vi "Save_file_txt_fifo.vi"(10 "传递队列":refnum<queue>, 11 "notifier":refnum<notifier>) -> ()   [LabVIEW 2012]
uses:
  <vilib>/GPower/VIRegister/Library/SubVIs/FindRegisterData.vi
  <vilib>/GPower/VIRegister/Library/SubVIs/WriteSub.vi
  <vilib>/GPower/Error/Library/FilterCodes.vi
  <vilib>/GPower/Error/Library/Filter/FilterMulti.vi
  <vilib>/GPower/VIRegister/Library/QManager/GetRegisterData.vi
  <vilib>/GPower/Error/Library/SetError.vi
  <vilib>/GPower/Error/Library/SplitAppended.vi
  <vilib>/GPower/VIRegister/Library/QManager/QManagerAction.vi
  <vilib>/GPower/Error/Library/ErrorType.vi
  <vilib>/GPower/Error/Library/SubVIs/ExplanationToError.vi
  <vilib>/GPower/VIRegister/Library/QManager/GetQName.vi
  <vilib>/GPower/VIRegister/Library/QManager/StartQManager.vi
  <vilib>/Utility/error.llb/Trim Whitespace.vi
  <vilib>/dlg_ctls.llb/Space Constant.vi
  <vilib>/Utility/error.llb/Error Code Database.vi
  <vilib>/GPower/Error/Library/SubVIs/SetStatus.vi
  <vilib>/GPower/Error/Library/AppendErrors.vi
  <vilib>/GPower/Error/Library/Append/AppendSingle.vi
  <vilib>/GPower/VIRegister/VIRegister.lvlib
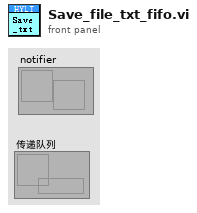
[diagram p1: front panel]
types:
  T1 = enum32{"invalid app kind", "Development System", "Run Time System", "Student Edition", "Embedded LabVIEW", "Evaluation", "Custom"}
  T2 = enum32{"Invalid", "Standard", "Closed", "Hidden", "Minimized", "Maximized"}
  T3 = enum16{"open", "replace", "create", "open or create", "replace or create", "replace or create with confirmation"}
  T4 = cluster{"Core":cluster{"Current VI Reference":refnum<vi>, "Close Panel on Exit?":bool}, "Zhufei":bool, "Your string data":string, "地检相位":i32, "file_Zhufen":refnum<file>, "notifier ":refnum<notifier>, "Beifen":bool, "file_Beifen":refnum<file>}
  T5 = cluster{"Current VI Reference":refnum<vi>, "Close Panel on Exit?":bool}
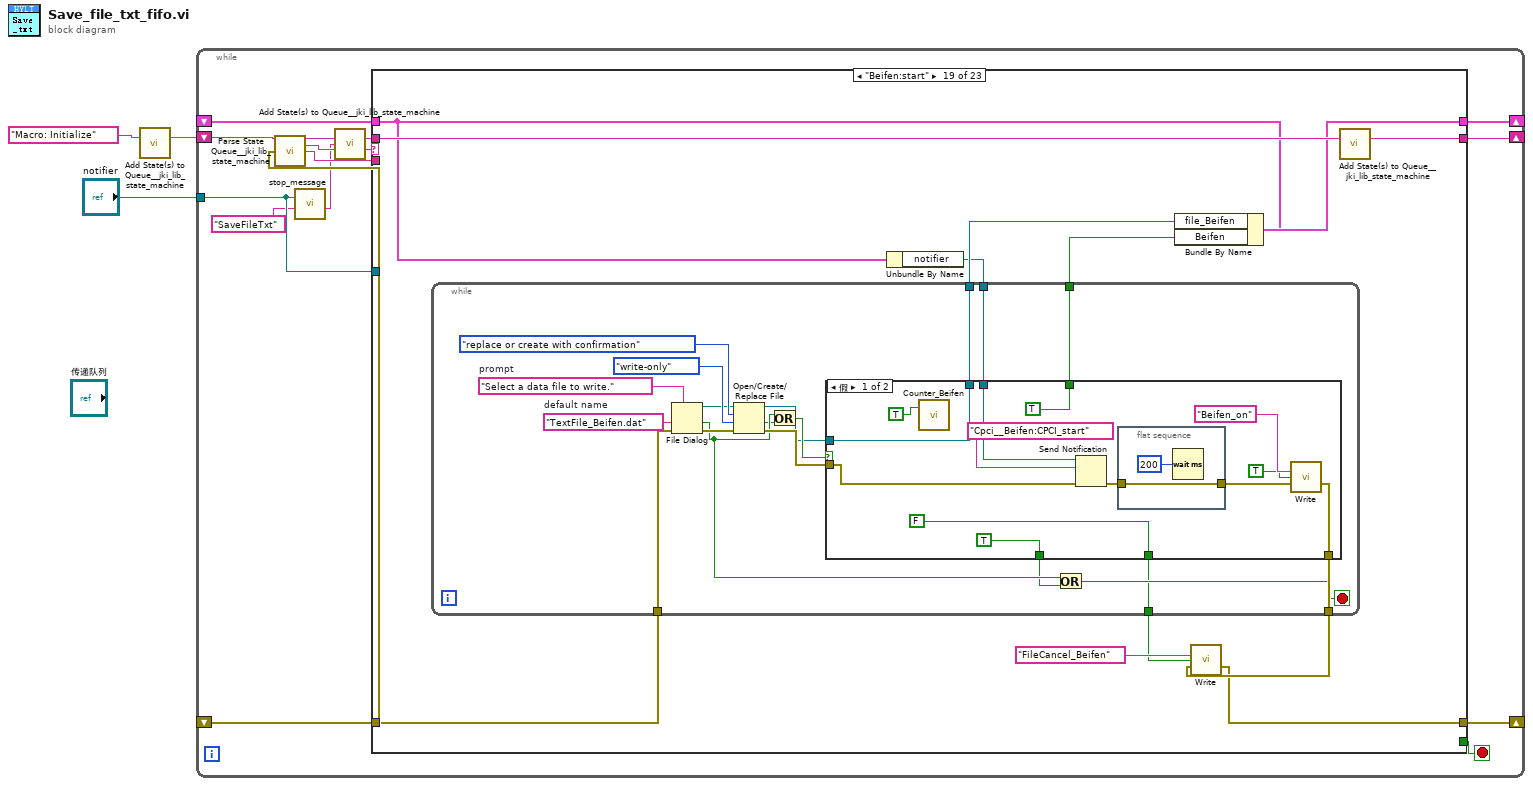
[diagram p0: block diagram]
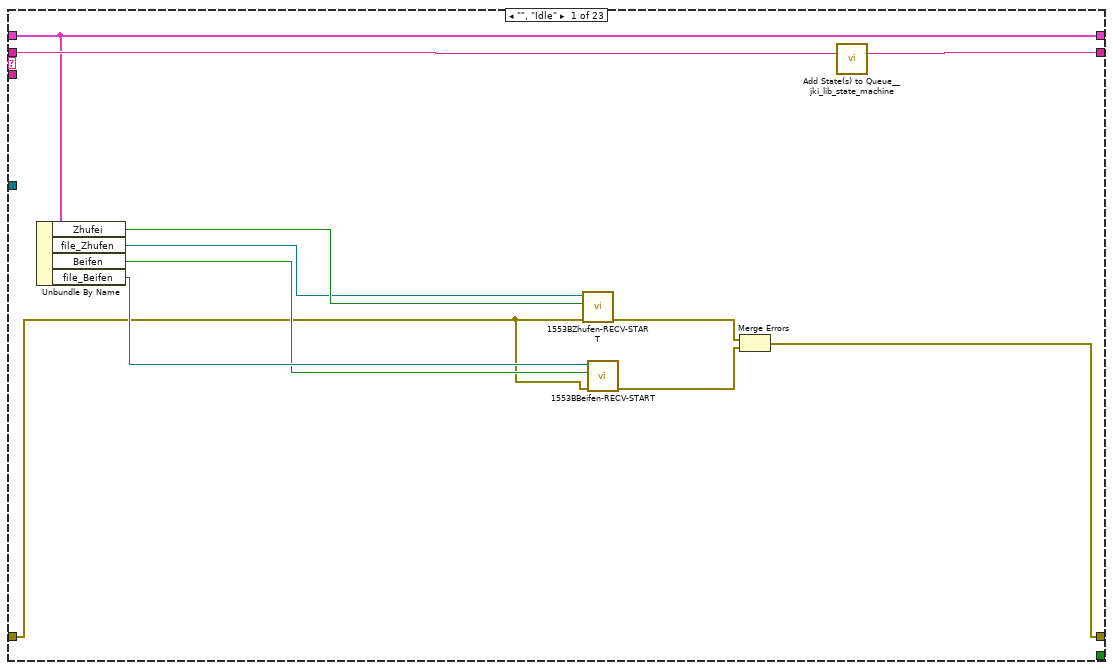
[diagram p2: hidden frame]
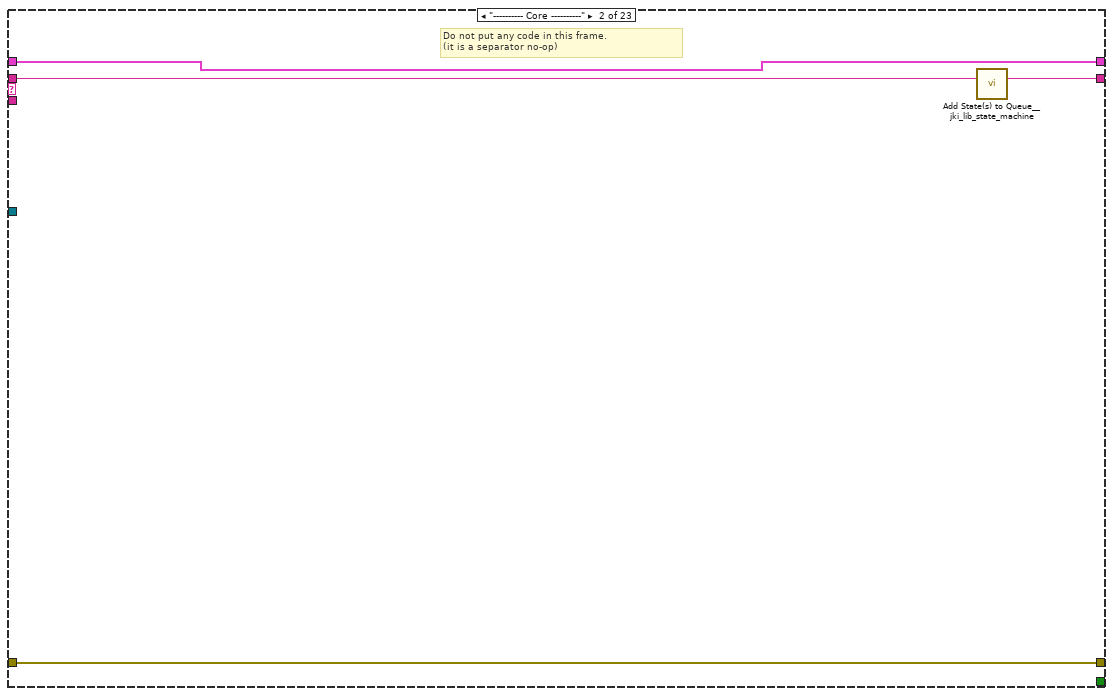
[diagram p3: hidden frame]
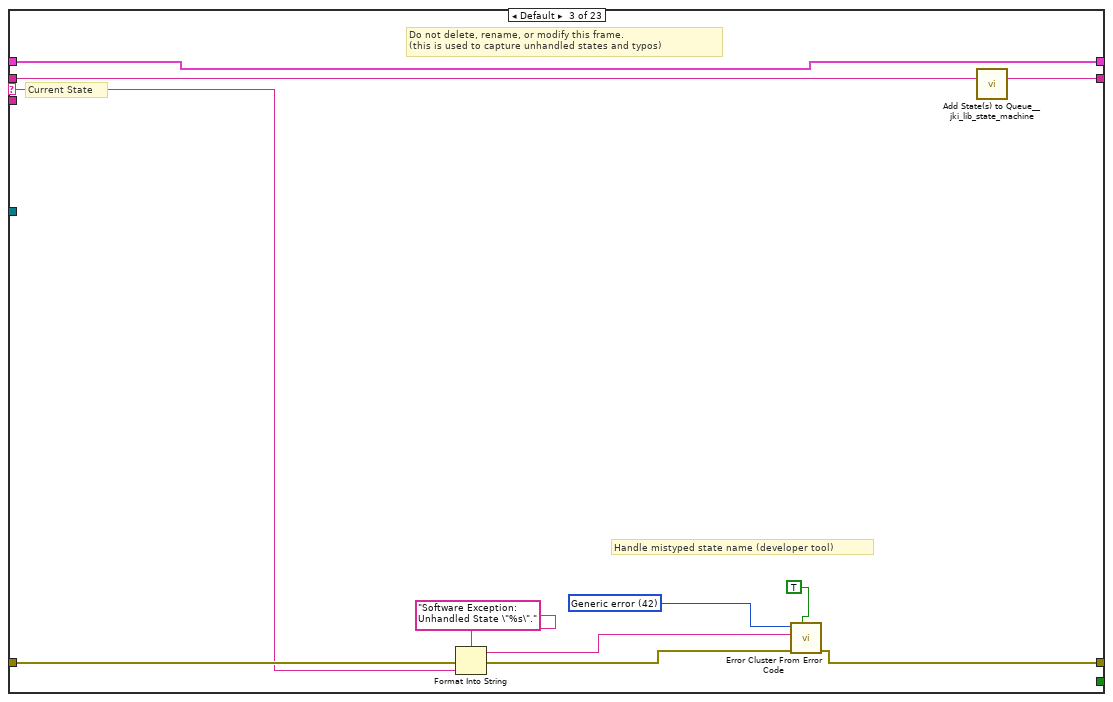
[diagram p4: hidden frame]
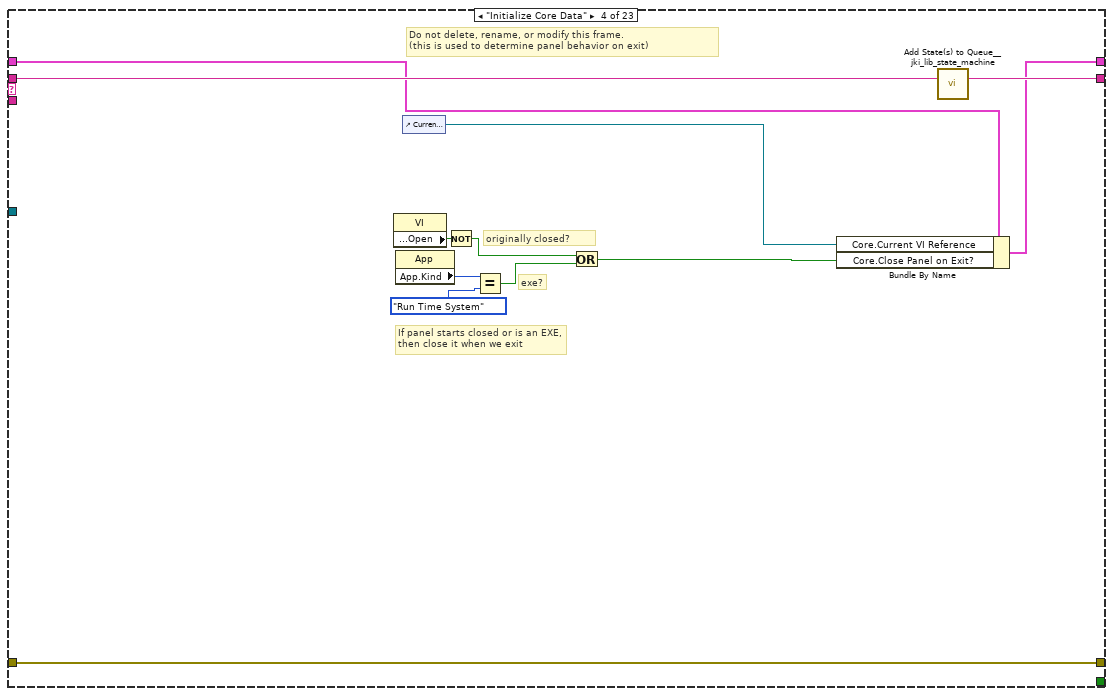
[diagram p5: hidden frame]
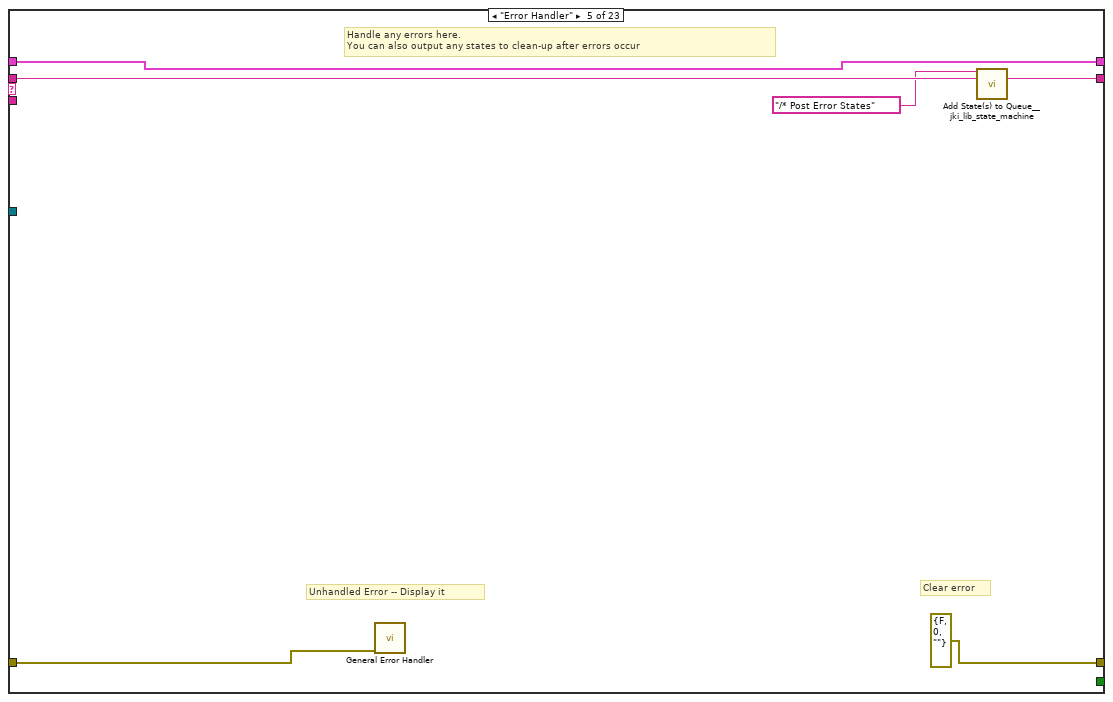
[diagram p6: hidden frame]
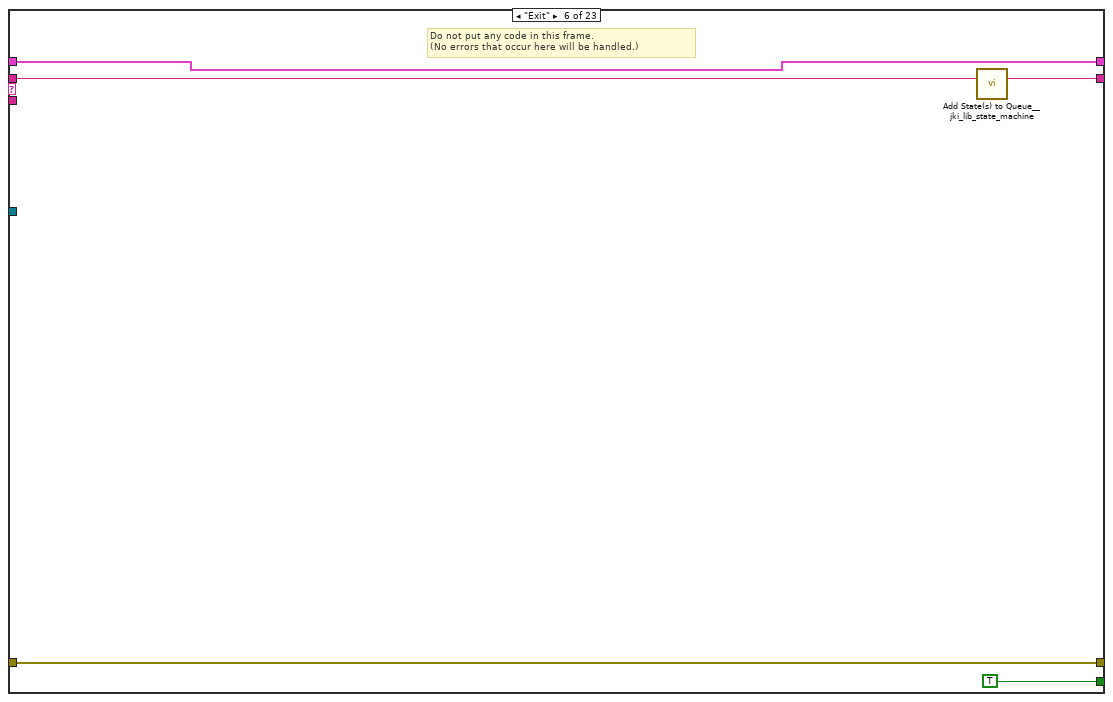
[diagram p7: hidden frame]
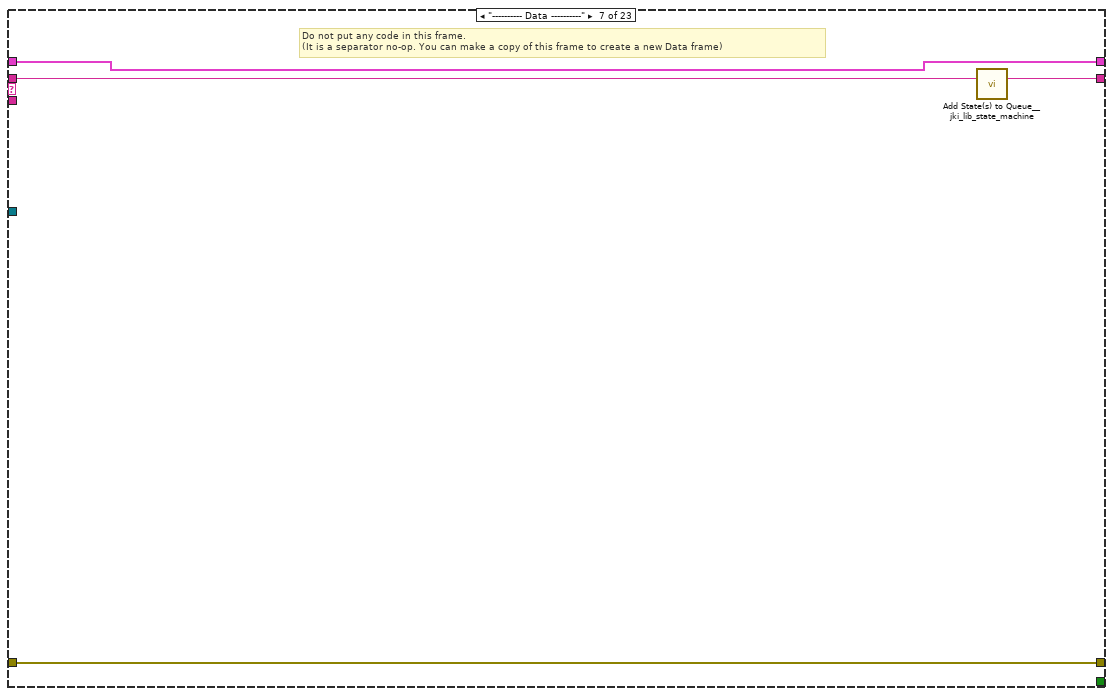
[diagram p8: hidden frame]
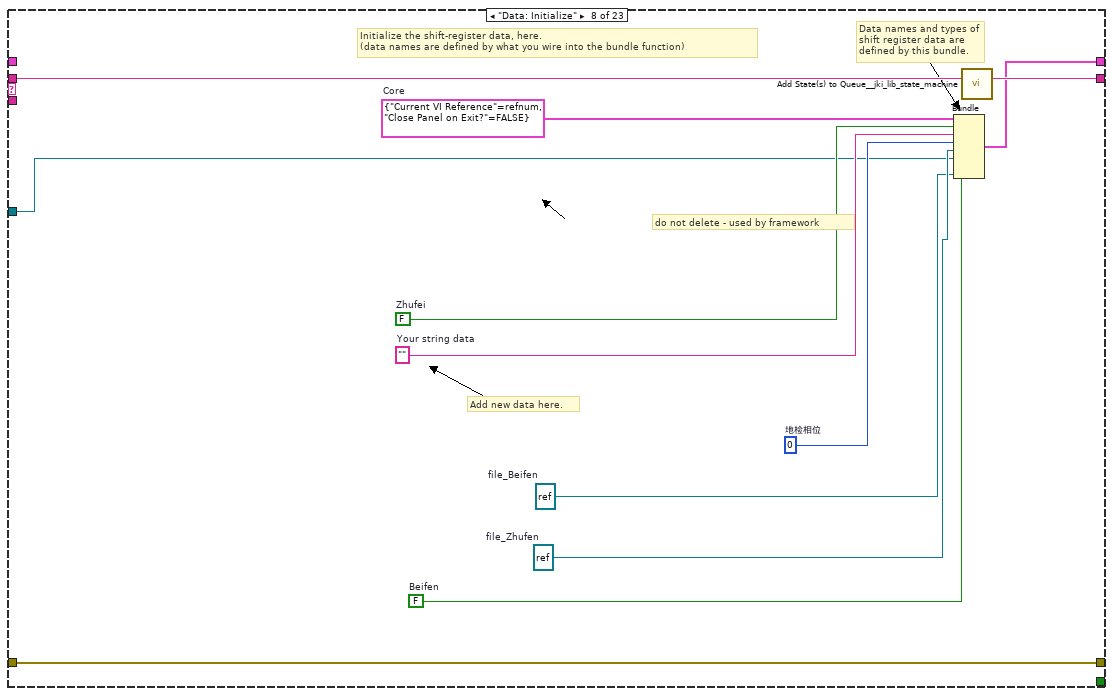
[diagram p9: hidden frame]
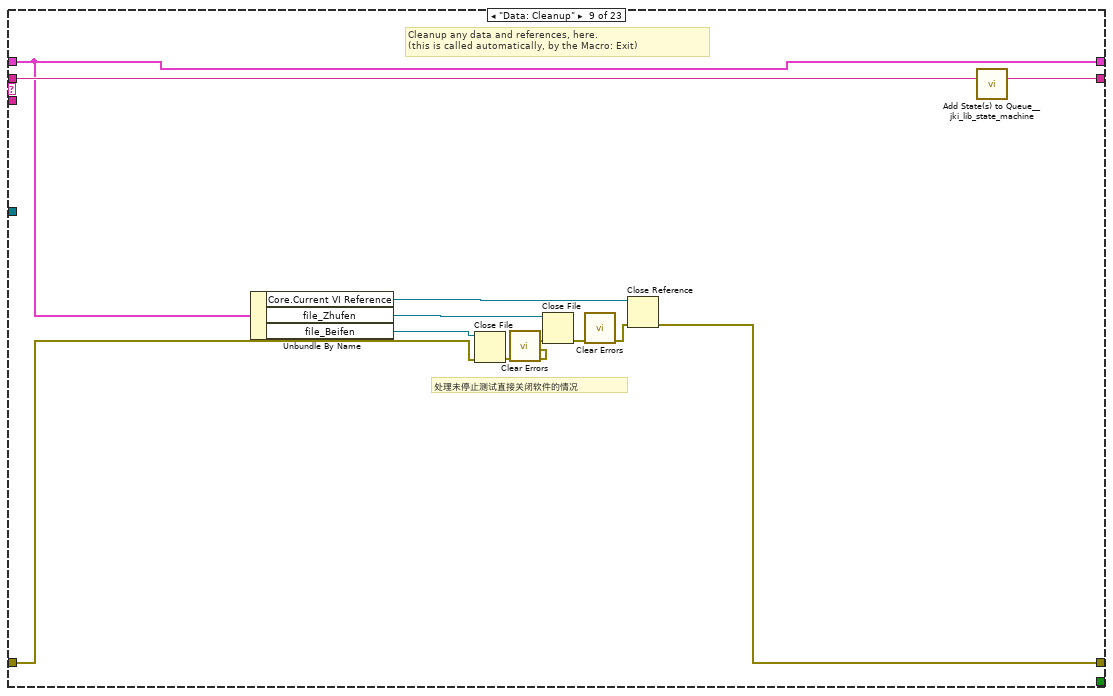
[diagram p10: hidden frame]
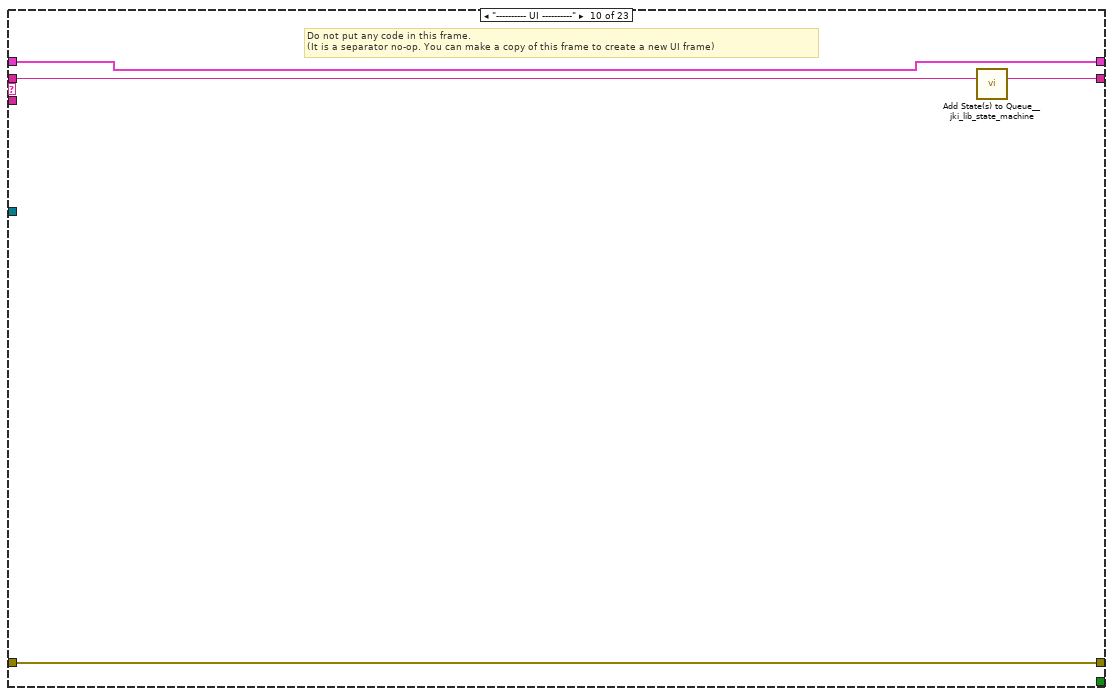
[diagram p11: hidden frame]
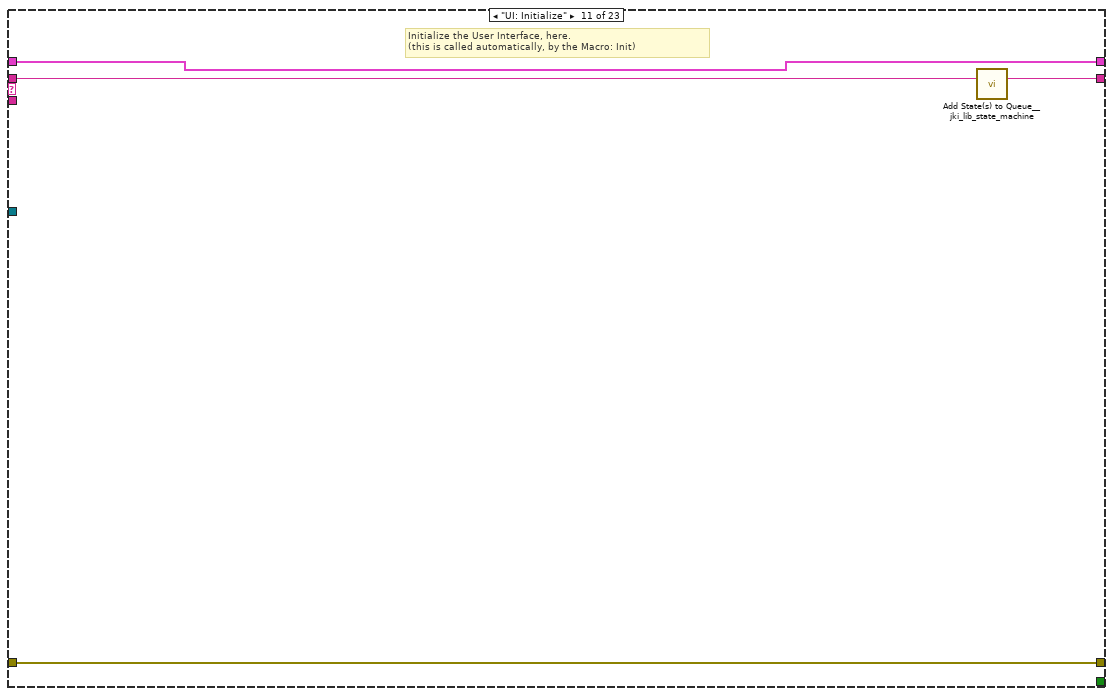
[diagram p12: hidden frame]
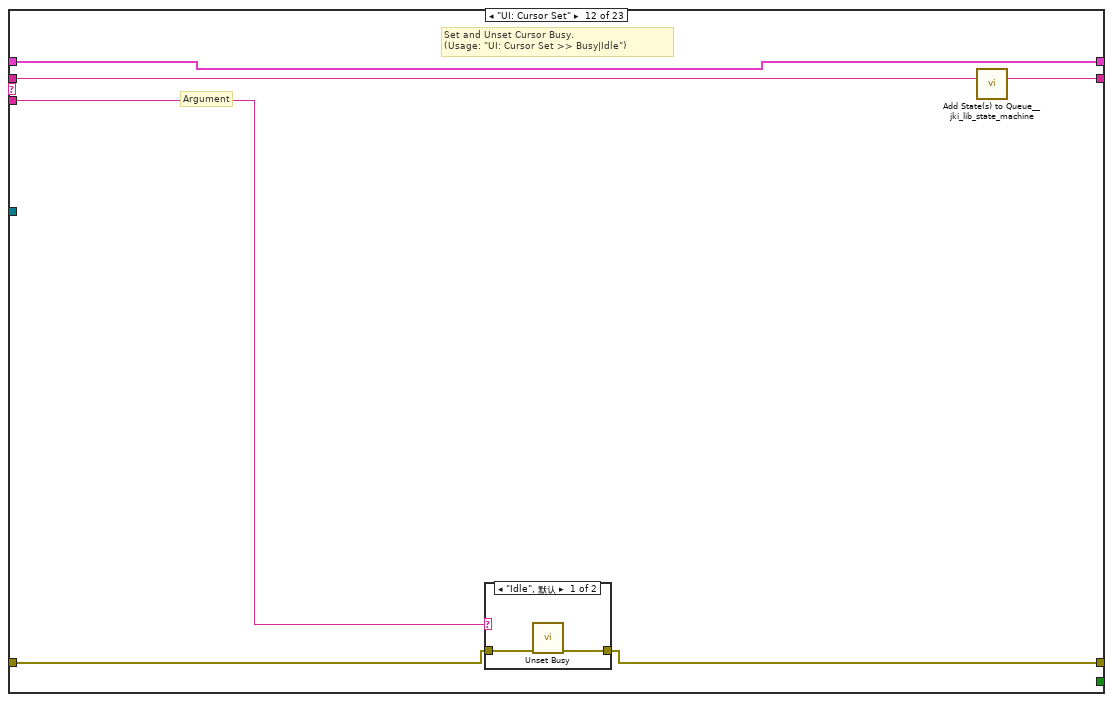
[diagram p13: hidden frame]
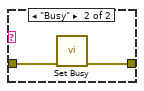
[diagram p14: hidden frame]
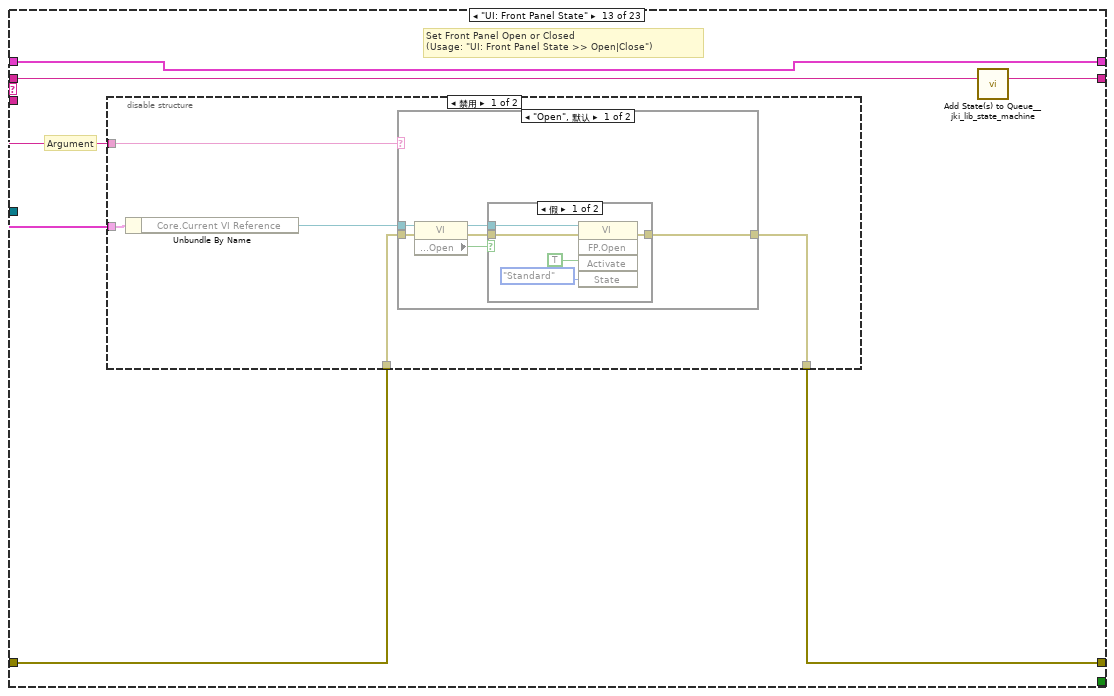
[diagram p15: hidden frame]
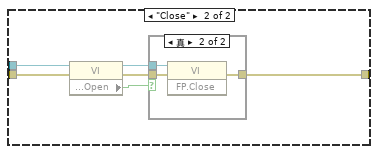
[diagram p17: hidden frame]
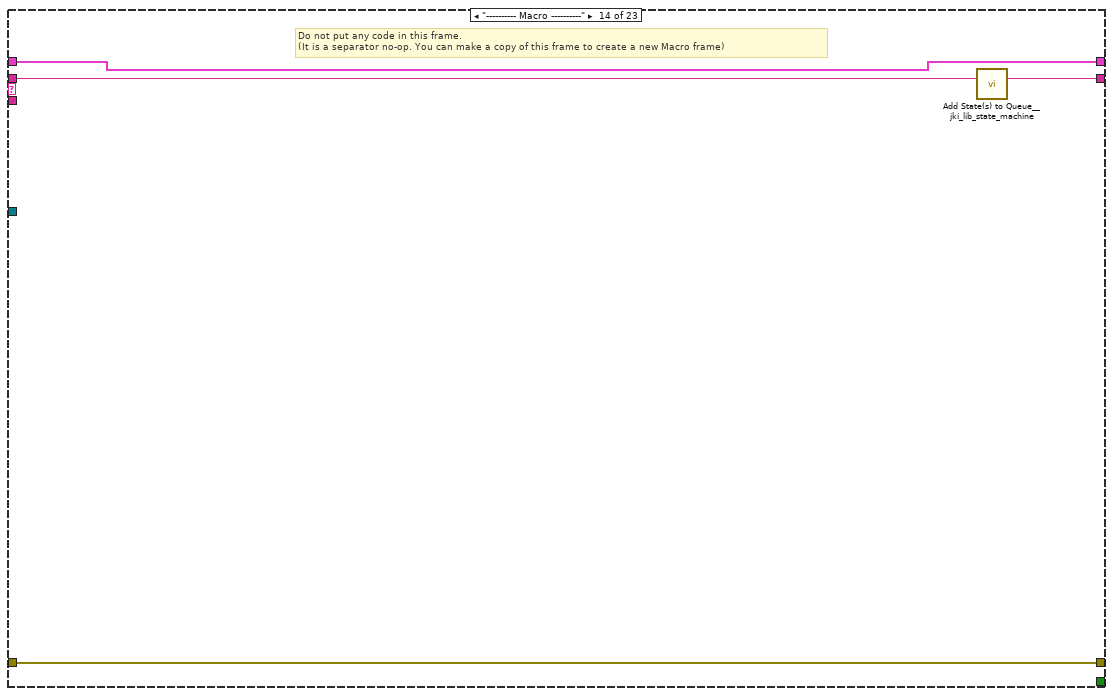
[diagram p20: hidden frame]
diagram:
  n1 = call <vilib>:"Add State(s) to Queue__jki_lib_state_machine.vi"("State(s) in (\"\")"="Macro: Initialize") -> ("States Out"=w3:string)  [unwired: 14 in]
  n2 = while "JKI - String-Based Queued State Machine (Basic) v1.0" {
    shift-right: [w11] -> _
    shift-left: _ -> [w10]
    shift-right: [w14] -> _
    shift-left: _ -> [w9]
    shift-right: [w13] -> _
    shift-left: w3 -> [w15]
    tunnel: "notifier" -> [w5]
    stop <- w12 stop-if-true
    n3 = call <vilib>:"Parse State Queue__jki_lib_state_machine.vi"("State Queue"=w15, "Error In (no error)"=w9) -> ("Remaining States"=w7:string, "Current State"=w17:string, "Arguments"=w16:string)  [unwired: 11 in]
    n4 = call "stop_message.vi"("识别符"="SaveFileTxt", "notifier"=w5) -> ("通知"=w6:string)  [unwired: 8 in, 1 out]
    n5 = call <vilib>:"Add State(s) to Queue__jki_lib_state_machine.vi"("State(s) in (\"\")"=w7, "State(s) at Back (\"\")"=w6) -> ("States Out"=w8:string)  [unwired: 13 in]
    n6 = case shown="\"Beifen:start\"" w17 {
      selector: w17 -> [_ _ w33 _ _ _ _ _ _ _ _ _ _ _ _ _ _ _ _ _ _ _ _]
      tunnel: w8 -> [w28 w32 w37 w55 w61 w66 w70 w82 w94 w98 w102 w108 w118 w149 w154 w164 w168 w180 w232 w282 w292 w296 w301]
      tunnel: w16 -> [_ _ _ _ _ _ _ _ _ _ _ w103 w113 _ _ _ _ _ _ _ _ _ _]
      tunnel: w10 -> [w26 w29 w35 w46 w58 w64 w67 _ w91 w95 w100 w106 w114 w146 w151 w161 w165 w174 w226 w277 w287 w293 w298]
      tunnel: [w24 w30 w39 w52 errorcluster {"status"=FALSE, "code"=0, "source"=""} ("error out") w63 w68 w79 w87 w96 w99 w104 w115 w147 w152 w162 w166 w169 w221 w273 w283 w294 w299] -> w14
      tunnel: w9 -> [w19 w30 w38 w52 w57 w63 w68 w79 w85 w96 w99 w105 w116 w147 w152 w162 w166 w175 w227 w279 w289 w294 w299]
      tunnel: [w27 w31 w36 w54 w60 w65 w69 w81 w93 w97 w101 w107 w117 w148 w153 w163 w167 w179 w231 w281 w291 w295 w300] -> w13
      tunnel: [_ _ _ _ _ TRUE _ _ _ _ _ _ _ _ _ _ _ _ _ _ _ _ _] -> w12
      tunnel: [w26 w29 w35 w53 w58 w64 w67 w80 w91 w95 w100 w106 w114 w146 w151 w161 w165 w177 w229 w276 w286 w293 w298] -> w11
      tunnel: w5 -> [_ _ _ _ _ _ _ w73 _ _ _ _ _ _ _ _ _ _ _ _ _ _ _]
      frame "", "Idle" {
        n7 = Unbundle By Name(w26) -> ("Zhufei"=w25:bool, "file_Zhufen"=w23:refnum<file>, "Beifen"=w20:bool, "file_Beifen"=w21:refnum<file>)
        n8 = call "1553BZhufen-RECV-START.vi"("错误输入（无错误）"=w19, "Zhufen"=w25, "字节流文件输入"=w23) -> ("错误输出"=w22:errorcluster)  [unwired: 8 in]
        n9 = call "1553BBeifen-RECV-START.vi"("错误输入（无错误）"=w19, "Beifen"=w20, "字节流文件输入"=w21) -> ("错误输出"=w18:errorcluster)  [unwired: 8 in]
        n10 = Merge Errors(w22, w18) -> (w24:errorcluster)
        n11 = call <vilib>:"Add State(s) to Queue__jki_lib_state_machine.vi"("State(s) in (\"\")"=w28) -> ("States Out"=w27:string)  [unwired: 14 in]
      }
      frame "---------- Core ----------" {
        # "Do not put any code in this frame.\n(it is a separator no-op)"
        n12 = call <vilib>:"Add State(s) to Queue__jki_lib_state_machine.vi"("State(s) in (\"\")"=w32) -> ("States Out"=w31:string)  [unwired: 14 in]
      }
      frame Default {
        w42 = 42 items=["No error", "Argument error", "Memory is full", "Out of zone", "End of file", "File already open", "Generic file I/O error", "File not found", "File permission error", "Disk is full", "Duplicate path", "Too many files open", "System feature not enabled", "Resource file not found", "Cannot add resource", "Resource not found", "Image not found", "Image memory error", "Pen does not exist", "Config type invalid", "Config token not found", "Config parse error", "Config memory error", "Bad external code format", "Bad external code offset", "External code not present", "Null window", "Destroy window error", "Null menu", "Print aborted", "Bad print record", "Print driver error", "Windows error during printing", "Memory error during printing", "Print dialog error", "Generic print error", "Invalid device refnum", "Device not found", "Device parameter error", "Device unit error", "Cannot open device", "Device call aborted", "Generic error", "Cancelled by user", "Object ID too low", "Object ID too high", "Object not in heap", "Unknown heap", "Unknown object (invalid DefProc)", "Unknown object (DefProc not in table)", "Message out of range", "Invalid (null) method", "Unknown message", "Manager call not supported", "Bad address", "Network operation in progress", "Network operation timed out", "Connection is busy", "Network attribute not supported", "Network error", "Address in use", "System out of memory", "Connection aborted", "Connection refused", "Not connected", "Already connected", "Connection closed", "Initialization error (interapplication manager)", "Bad occurrence", "Wait on unbound occurrence handler", "Occurrence queue overflow", "Datalog type conflict", "Unused", "Unrecognized type (interapplication manager)", "Memory corrupt", "Failed to make temporary DLL", "Old CIN version", "Drag socket not found", "Failed to load drop-object", "Failed to register OLE object", "Failed to release OLE object", "Format specifier type mismatch", "Unknown format specifier", "Too few format specifiers", "Too many format specifiers", "Scan failed", "Newer CIN version", "Error converting to variant", "Runtime menu error", "Password tampered", "Variant attribute not found", "Incompatible variant data type", "Event data is not available", "Event Store is not present", "Occurrence is not found", "Event Queue is not created", "Event info is not available", "Refnum passed is NULL", "Error retrieving Class GUID", "Error retrieving CoClass GUID", "Error retrieving TypeLib GUID.", "Bad built application magic bytes.", "Specific driver is different from the specific driver associated with the Logical Name.", "There is no session opened to the class driver.", "Max Error", "MAX - Error with config objects", "MAX - Error loading configuration", "MAX - Group not supported"]
        # "Current State"
        # "Do not delete, rename, or modify this frame.\n(this is used to capture unhandled states and typos)"
        # "Handle mistyped state name (developer tool)"
        n13 = Format Into String(format string="Software Exception: Unhandled State \"%s\"." ("message"), error in=w38, w33) -> (resulting string=w41:string, error out=w40:errorcluster)  [unwired: 1 in]
        n14 = call <vilib>:"Error Cluster From Error Code.vi"("show call chain? (False)"=TRUE, "error in (no error)"=w40, "error message (\"\")"=w41, "error code (0)"=w42) -> ("error out"=w39:errorcluster)  [unwired: 5 in]
        n15 = call <vilib>:"Add State(s) to Queue__jki_lib_state_machine.vi"("State(s) in (\"\")"=w37) -> ("States Out"=w36:string)  [unwired: 14 in]
      }
      frame "Initialize Core Data" {
        # "Do not delete, rename, or modify this frame.\n(this is used to determine panel behavior on exit)"
        # "originally closed?"
        # "exe?"
        # "If panel starts closed or is an EXE, then close it when we exit"
        n16 = property class="VI"() -> ("Front Panel.Open"=w51:bool)  [unwired: 2 in, 2 out]
        n17 = property class="App"() -> ("App.Kind"=w50:T1)  [unwired: 2 in, 2 out]
        n18 = control-ref of="Current VI Reference"() -> (w44:refnum<vi>)
        n19 = Not(x=w51) -> (.not. x?=w48:bool)
        n20 = Equal?(x=w50, y=T1."Run Time System" ("Application:Kind")) -> (x = y?=w47:bool)
        n21 = Or(x=w48, y=w47) -> (x .or. y?=w45:bool)
        n22 = Bundle By Name(cluster=w46, "Core.Current VI Reference"=w44, "Core.Close Panel on Exit?"=w45) -> (w53:T4)
        n23 = call <vilib>:"Add State(s) to Queue__jki_lib_state_machine.vi"("State(s) in (\"\")"=w55) -> ("States Out"=w54:string)  [unwired: 14 in]
      }
      frame "Error Handler" {
        # "Unhandled Error -- Display it"
        # "Handle any errors here.\nYou can also output any states to clean-up after errors occur"
        # "Clear error"
        n24 = call <vilib>:"General Error Handler.vi"("error in (no error)"=w57) -> ()  [unwired: 10 in, 5 out]
        n25 = call <vilib>:"Add State(s) to Queue__jki_lib_state_machine.vi"("State(s) in Front (\"\")"="/* Post Error States", "State(s) in (\"\")"=w61) -> ("States Out"=w60:string)  [unwired: 13 in]
      }
      frame "Exit" {
        # "Do not put any code in this frame.\n(No errors that occur here will be handled.)"
        n26 = call <vilib>:"Add State(s) to Queue__jki_lib_state_machine.vi"("State(s) in (\"\")"=w66) -> ("States Out"=w65:string)  [unwired: 14 in]
      }
      frame "---------- Data ----------" {
        # "Do not put any code in this frame.\n(It is a separator no-op. You can make a copy of this frame to create a new Data frame)"
        n27 = call <vilib>:"Add State(s) to Queue__jki_lib_state_machine.vi"("State(s) in (\"\")"=w70) -> ("States Out"=w69:string)  [unwired: 14 in]
      }
      frame "Data: Initialize" {
        w71 = refnum<file> refnum  # file_Beifen
        w72 = FALSE  # Beifen
        w74 = refnum<file> refnum  # file_Zhufen
        w75 = 0  # 地检相位
        w76 = T5 {"Current VI Reference"=refnum, "Close Panel on Exit?"=FALSE}  # Core
        w78 = FALSE  # Zhufei
        w77 = ""  # Your string data
        # "do not delete - used by framework"
        # "Add new data here."
        # "Data names and types of shift register data are defined by this bundle."
        # "Initialize the shift-register data, here.\n(data names are defined by what you wire into the bundle function)"
        n28 = Bundle("Core"=w76, "Zhufei"=w78, "Your string data"=w77, "地检相位"=w75, "file_Zhufen"=w74, "notifier"=w73, "Beifen"=w72, "file_Beifen"=w71) -> (w80:T4)  [unwired: 1 in]
        n29 = call <vilib>:"Add State(s) to Queue__jki_lib_state_machine.vi"("State(s) in (\"\")"=w82) -> ("States Out"=w81:string)  [unwired: 14 in]
      }
      frame "Data: Cleanup" {
        # "处理未停止测试直接关闭软件的情况"
        # "Cleanup any data and references, here.\n(this is called automatically, by the Macro: Exit)"
        n30 = Unbundle By Name(w91) -> ("Core.Current VI Reference"=w92:refnum<vi>, "file_Zhufen"=w90:refnum<file>, "file_Beifen"=w86:refnum<file>)
        n31 = Close File(refnum=w86, error in=w85) -> (error out=w83:errorcluster)  [unwired: 1 out]
        n32 = call <vilib>:"Clear Errors.vi"("error in (no error)"=w83) -> ("error out"=w84:errorcluster)  [unwired: 6 in]
        n33 = Close File(refnum=w90, error in=w84) -> (error out=w89:errorcluster)  [unwired: 1 out]
        n34 = call <vilib>:"Clear Errors.vi"("error in (no error)"=w89) -> ("error out"=w88:errorcluster)  [unwired: 6 in]
        n35 = Close Reference(reference=w92, error in (no error)=w88) -> (error out=w87:errorcluster)
        n36 = call <vilib>:"Add State(s) to Queue__jki_lib_state_machine.vi"("State(s) in (\"\")"=w94) -> ("States Out"=w93:string)  [unwired: 14 in]
      }
      frame "---------- UI ----------" {
        # "Do not put any code in this frame.\n(It is a separator no-op. You can make a copy of this frame to create a new UI frame)"
        n37 = call <vilib>:"Add State(s) to Queue__jki_lib_state_machine.vi"("State(s) in (\"\")"=w98) -> ("States Out"=w97:string)  [unwired: 14 in]
      }
      frame "UI: Initialize" {
        # "Initialize the User Interface, here.\n(this is called automatically, by the Macro: Init)"
        n38 = call <vilib>:"Add State(s) to Queue__jki_lib_state_machine.vi"("State(s) in (\"\")"=w102) -> ("States Out"=w101:string)  [unwired: 14 in]
      }
      frame "UI: Cursor Set" {
        # "Argument"
        # "Set and Unset Cursor Busy.\n(Usage: \"UI: Cursor Set >> Busy|Idle\")"
        n39 = case shown="\"Idle\", 默认" w103 {
          tunnel: w105 -> [w110 w112]
          tunnel: [w109 w111] -> w104
          frame "Idle", Default {
            n40 = call <vilib>:"Unset Busy.vi"("error in (no error)"=w110) -> ("error out"=w109:errorcluster)  [unwired: 10 in]
          }
          frame "Busy" {
            n41 = call <vilib>:"Set Busy.vi"("error in (no error)"=w112) -> ("error out"=w111:errorcluster)  [unwired: 9 in, 1 out]
          }
        }
        n42 = call <vilib>:"Add State(s) to Queue__jki_lib_state_machine.vi"("State(s) in (\"\")"=w108) -> ("States Out"=w107:string)  [unwired: 14 in]
      }
      frame "UI: Front Panel State" {
        # "Argument"
        # "Set Front Panel Open or Closed\n(Usage: \"UI: Front Panel State >> Open|Close\")"
        n43 = disable-structure shown="禁用" {
          disable-tunnel: w116 -> [w123 _]
          disable-tunnel: [w122 _] -> w115
          disable-tunnel: w114 -> [w121 _]
          disable-tunnel: w113 -> [w119 _]
          frame Disabled {
            n44 = Unbundle By Name(w121) -> ("Core.Current VI Reference"=w120:refnum<vi>)
            n45 = case shown="\"Open\", 默认" w119 {
              tunnel: w123 -> [w127 w140]
              tunnel: [w129 w141] -> w122
              tunnel: w120 -> [w128 w138]
              frame "Open", Default {
                n46 = property class="VI"(reference=w128, error in=w127) -> (reference out=w125:refnum<vi>, error out=w126:errorcluster, "Front Panel.Open"=w124:bool)
                n47 = case shown="假" w124 {
                  tunnel: [w132 w135] -> w129
                  tunnel: w126 -> [w131 w135]
                  tunnel: w125 -> [w130 _]
                  frame False {
                    n48 = invoke class="VI" method="FP.Open"(reference=w130, error in=w131, "Activate"=TRUE, "State"=T2."Standard") -> (error out=w132:errorcluster)  [unwired: 1 in, 4 out]
                  }
                  frame True {
                  }
                }
              }
              frame "Close" {
                n49 = property class="VI"(reference=w138, error in=w140) -> (reference out=w137:refnum<vi>, error out=w139:errorcluster, "Front Panel.Open"=w136:bool)
                n50 = case shown="真" w136 {
                  tunnel: [w142 w145] -> w141
                  tunnel: w139 -> [w142 w144]
                  tunnel: w137 -> [_ w143]
                  frame False {
                  }
                  frame True {
                    n51 = invoke class="VI" method="FP.Close"(reference=w143, error in=w144) -> (error out=w145:errorcluster)  [unwired: 1 in, 2 out]
                  }
                }
              }
            }
          }
          frame Enabled {
          }
        }
        n52 = call <vilib>:"Add State(s) to Queue__jki_lib_state_machine.vi"("State(s) in (\"\")"=w118) -> ("States Out"=w117:string)  [unwired: 14 in]
      }
      frame "---------- Macro ----------" {
        # "Do not put any code in this frame.\n(It is a separator no-op. You can make a copy of this frame to create a new Macro frame)"
        n53 = call <vilib>:"Add State(s) to Queue__jki_lib_state_machine.vi"("State(s) in (\"\")"=w149) -> ("States Out"=w148:string)  [unwired: 14 in]
      }
      frame "Macro: Initialize" {
        w150 = "Data: Initialize\nInitialize Core Data\nUI: Initialize\nUI: Front Panel State >> Open"  # Data: Initialize Initialize Core Data UI: Initialize UI: Front Panel State >> Open
        # "Initialization Macro\n(This is called once, when the VI starts)"
        n54 = call <vilib>:"Add State(s) to Queue__jki_lib_state_machine.vi"("State(s) in Front (\"\")"=w150, "State(s) in (\"\")"=w154) -> ("States Out"=w153:string)  [unwired: 13 in]
      }
      frame "Macro: Exit" {
        # "Exit Macro\n(This is called once, when the VI exits)"
        n55 = Unbundle By Name(w161) -> ("Core.Close Panel on Exit?"=w160:bool)
        n56 = Select(t="UI: Front Panel State >> Close", s=w160, f="") -> (s? t:f=w157:string)
        n57 = call <vilib>:"Add State(s) to Queue__jki_lib_state_machine.vi"("State(s) in (\"\")"=w157, "State(s) at Back (\"\")"="Data: Cleanup\nExit") -> ("States Out"=w155:string)  [unwired: 13 in]
        n58 = call <vilib>:"Add State(s) to Queue__jki_lib_state_machine.vi"("State(s) in Front (\"\")"=w155, "State(s) in (\"\")"=w164) -> ("States Out"=w163:string)  [unwired: 13 in]
      }
      frame "---------- Zhufen ----------" {
        # "Template Separator\n(You can make a copy of, or modify, this frame)"
        n59 = call <vilib>:"Add State(s) to Queue__jki_lib_state_machine.vi"("State(s) in (\"\")"=w168) -> ("States Out"=w167:string)  [unwired: 14 in]
      }
      frame "Zhufen:start" {
        n60 = Unbundle By Name(w174) -> ("notifier"=w173:refnum<notifier>)
        n61 = while {
          tunnel: [w197] -> w178
          tunnel: [w196] -> w176
          tunnel: w175 -> [w195]
          tunnel: w173 -> [w194]
          tunnel: [w193] -> w170
          tunnel: [w181] -> w171
          stop <- w182 stop-if-true
          w199 = "TextFile.dat"  # default name
          w198 = "Select a data file to write."  # prompt
          n62 = File Dialog(7:w198, 8:w195, 9:w199) -> (0:w189:errorcluster, 1:w185:bool, 3:w187:path)  [unwired: 5 out]
          n63 = Open/Create/Replace File(file path (use dialog)=w187, error in=w189, operation (0:open)=T3."replace or create with confirmation", access (0:read/write)=enum16{"read/write", "read-only", "write-only"}."write-only") -> (refnum out=w186:refnum<file>, cancelled=w184:bool, error out=w188:errorcluster)  [unwired: 2 out]
          n64 = Or(x=w185, y=w184) -> (x .or. y?=w190:bool)
          n65 = case shown="假" w190 {
            tunnel: w186 -> [w204 _]
            tunnel: w188 -> [w203 w218]
            tunnel: [w204 refnum<file> refnum ("refnum out")] -> w197
            tunnel: [TRUE ("Your Boolean data") FALSE ("Your Boolean data")] -> w196
            tunnel: w194 -> [w208 _]
            tunnel: [w205 w217] -> w193
            tunnel: [TRUE FALSE] -> w183
            tunnel: [FALSE TRUE] -> w181
            frame False {
              n66 = call "Counter.vi"("Reset(F)"=TRUE) -> ()  [unwired: 1 out]
              n67 = Send Notification(notification="Cpci__Zhufen:CPCI_start" ("通知"), notifier=w208, error in (no error)=w203) -> (error out=w207:errorcluster)  [unwired: 1 out]
              n68 = flat-sequence {
                tunnel: w207 -> [w213]
                tunnel: [w213] -> w206
                frame #0 {
                  n69 = Wait (ms)(milliseconds to wait=u32 200 ("等待时间（毫秒）")) -> ()  [unwired: 1 out]
                }
              }
              n70 = call <vilib>:"Write.vi"("Register name"="Zhufen_on", "Register value"=TRUE ("开始测量"), "Error in"=w206) -> ("Error out"=w205:errorcluster)  [unwired: 10 in, 2 out]
            }
            frame True {
              n71 = call <vilib>:"Clear Errors.vi"("error in (no error)"=w218) -> ("error out"=w217:errorcluster)  [unwired: 6 in]
            }
          }
          n72 = Or(x=w185, y=w183) -> (x .or. y?=w182:bool)
        }
        n73 = Bundle By Name(cluster=w174, "file_Zhufen"=w178, "Zhufei"=w176) -> (w177:T4)
        n74 = call <vilib>:"Write.vi"("Register name"="FileCancel", "Register value"=w171, "Error in"=w170) -> ("Error out"=w169:errorcluster)  [unwired: 10 in, 2 out]
        n75 = call <vilib>:"Add State(s) to Queue__jki_lib_state_machine.vi"("State(s) in (\"\")"=w180) -> ("States Out"=w179:string)  [unwired: 14 in]
      }
      frame "Beifen:start" {
        n76 = Unbundle By Name(w226) -> ("notifier"=w225:refnum<notifier>)
        n77 = while {
          tunnel: [w249] -> w230
          tunnel: [w248] -> w228
          tunnel: w227 -> [w247]
          tunnel: w225 -> [w246]
          tunnel: [w245] -> w222
          tunnel: [w233] -> w223
          stop <- w234 stop-if-true
          w251 = "TextFile_Beifen.dat"  # default name
          w250 = "Select a data file to write."  # prompt
          n78 = File Dialog(7:w250, 8:w247, 9:w251) -> (0:w241:errorcluster, 1:w237:bool, 3:w239:path)  [unwired: 5 out]
          n79 = Open/Create/Replace File(file path (use dialog)=w239, error in=w241, operation (0:open)=T3."replace or create with confirmation", access (0:read/write)=enum16{"read/write", "read-only", "write-only"}."write-only") -> (refnum out=w238:refnum<file>, cancelled=w236:bool, error out=w240:errorcluster)  [unwired: 2 out]
          n80 = Or(x=w237, y=w236) -> (x .or. y?=w242:bool)
          n81 = case shown="假" w242 {
            tunnel: w238 -> [w256 _]
            tunnel: w240 -> [w255 w270]
            tunnel: [w256 refnum<file> refnum ("refnum out")] -> w249
            tunnel: [TRUE ("Your Boolean data") FALSE ("Your Boolean data")] -> w248
            tunnel: w246 -> [w260 _]
            tunnel: [w257 w269] -> w245
            tunnel: [TRUE FALSE] -> w235
            tunnel: [FALSE TRUE] -> w233
            frame False {
              n82 = call "Counter_Beifen.vi"("Reset(F)"=TRUE) -> ()  [unwired: 2 in, 1 out]
              n83 = Send Notification(notification="Cpci__Beifen:CPCI_start" ("通知"), notifier=w260, error in (no error)=w255) -> (error out=w259:errorcluster)  [unwired: 1 out]
              n84 = flat-sequence {
                tunnel: w259 -> [w265]
                tunnel: [w265] -> w258
                frame #0 {
                  n85 = Wait (ms)(milliseconds to wait=u32 200 ("等待时间（毫秒）")) -> ()  [unwired: 1 out]
                }
              }
              n86 = call <vilib>:"Write.vi"("Register name"="Beifen_on", "Register value"=TRUE ("开始测量"), "Error in"=w258) -> ("Error out"=w257:errorcluster)  [unwired: 10 in, 2 out]
            }
            frame True {
              n87 = call <vilib>:"Clear Errors.vi"("error in (no error)"=w270) -> ("error out"=w269:errorcluster)  [unwired: 6 in]
            }
          }
          n88 = Or(x=w237, y=w235) -> (x .or. y?=w234:bool)
        }
        n89 = Bundle By Name(cluster=w226, "file_Beifen"=w230, "Beifen"=w228) -> (w229:T4)
        n90 = call <vilib>:"Write.vi"("Register name"="FileCancel_Beifen", "Register value"=w223, "Error in"=w222) -> ("Error out"=w221:errorcluster)  [unwired: 10 in, 2 out]
        n91 = call <vilib>:"Add State(s) to Queue__jki_lib_state_machine.vi"("State(s) in (\"\")"=w232) -> ("States Out"=w231:string)  [unwired: 14 in]
      }
      frame "Zhufen:stop" {
        # "Your code here.\n(You can make a copy of, or modify, this frame)"
        n92 = Unbundle By Name(w277) -> ("file_Zhufen"=w280:refnum<file>)
        n93 = Close File(refnum=w280, error in=w279) -> (error out=w275:errorcluster)  [unwired: 1 out]
        n94 = call <vilib>:"EmptyBuffer.vi"("Register name"="1553BZhuFenRecv", "Error in"=w275) -> ("Error out"=w273:errorcluster)  [unwired: 11 in, 2 out]
        n95 = Bundle By Name(cluster=w277, "Zhufei"=FALSE ("Your Boolean data")) -> (w276:T4)
        n96 = call <vilib>:"Add State(s) to Queue__jki_lib_state_machine.vi"("State(s) in (\"\")"=w282) -> ("States Out"=w281:string)  [unwired: 14 in]
      }
      frame "Beifen:stop" {
        # "Your code here.\n(You can make a copy of, or modify, this frame)"
        n97 = Unbundle By Name(w287) -> ("file_Beifen"=w290:refnum<file>)
        n98 = Close File(refnum=w290, error in=w289) -> (error out=w285:errorcluster)  [unwired: 1 out]
        n99 = call <vilib>:"EmptyBuffer.vi"("Register name"="1553BBeiFenRecv", "Error in"=w285) -> ("Error out"=w283:errorcluster)  [unwired: 11 in, 2 out]
        n100 = Bundle By Name(cluster=w287, "Beifen"=FALSE ("Your Boolean data")) -> (w286:T4)
        n101 = call <vilib>:"Add State(s) to Queue__jki_lib_state_machine.vi"("State(s) in (\"\")"=w292) -> ("States Out"=w291:string)  [unwired: 14 in]
      }
      frame "---------- Exit ----------" {
        # "Template Separator\n(You can make a copy of, or modify, this frame)"
        n102 = call <vilib>:"Add State(s) to Queue__jki_lib_state_machine.vi"("State(s) in (\"\")"=w296) -> ("States Out"=w295:string)  [unwired: 14 in]
      }
      frame "Exit:all" {
        # "Your code here.\n(You can make a copy of, or modify, this frame)"
        n103 = call <vilib>:"Add State(s) to Queue__jki_lib_state_machine.vi"("State(s) in Front (\"\")"="Macro: Exit" ("State(s) in Front (\"\")"), "State(s) in (\"\")"=w301) -> ("States Out"=w300:string)  [unwired: 13 in]
      }
    }
  }
